vi "CD Init_Prepare Inline Data_Fill In BC part of Frame Descriptor.vi"(11 "message":T5 {"Timestamp Channel Data Reference" format="%.0x"; "Status Channel Data Refs" format="%.0x"; "Words Item Refs" format="%.0x"; "Words Block Data Refs"."Data Reference" format="%.0x"}) -> (3 "BC Frame Descriptor":T1 {"Status Channel Refs" format="%.0x"; "Words Block Data Refs"."Data Reference" format="%.0x"; "Timestamp Channel Data Reference" format="%.0x"})   [LabVIEW 2017, in "Ballard MIL-1553 Engine.lvlib"]
uses:
  Ballard MIL-1553 Engine.lvlib
  Shared/Controls and Global/RT Message.ctl
  Shared/Controls and Global/RT messageType.ctl
  Shared/Controls and Global/RT CWD1.ctl
  Shared/Controls and Global/RT CWD2.ctl
  <vilib>/NI Veristand/Custom Device API/Data Reference.ctl
  <vilib>/NI Veristand/Custom Device API/Custom Device Item Ref.ctl
  <vilib>/NI Veristand/Custom Device API/Block Data Reference.ctl
  Controls/RT Inline Frame Descriptor_BC.ctl
  <vilib>/NI VeriStand/Custom Device API/Custom Device API.lvlib
  Shared/Ballard 1553 Shared.lvlib
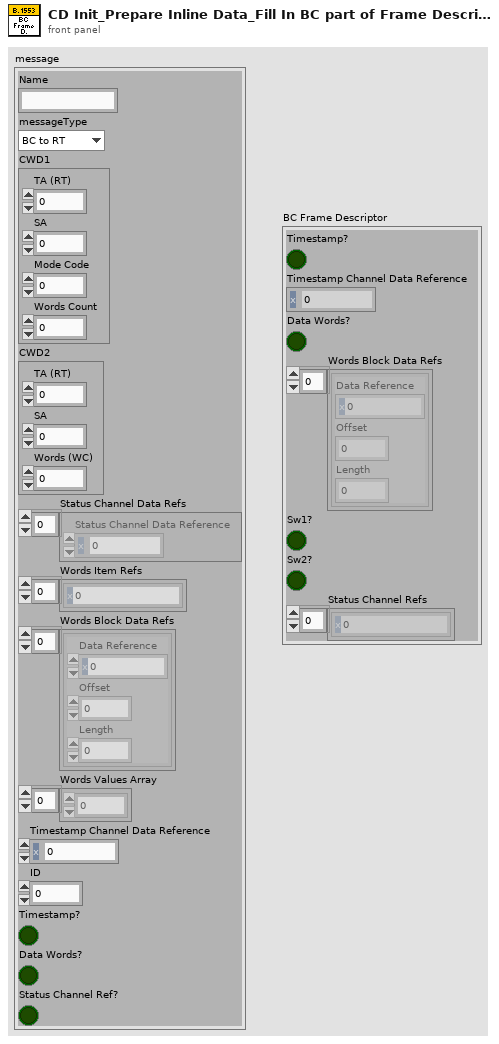
[diagram p1: front panel]
types:
  T1 = typedef "Ballard MIL-1553 Engine.lvlib/RT Inline Frame Descriptor_BC.ctl" = cluster{"Timestamp?":bool, "Timestamp Channel Data Reference":T2, "Data Words?":bool, "Words Block Data Refs":T3[], "Sw1?":bool, "Sw2?":bool, "Status Channel Refs":T4[]}
  T2 = typedef "Custom Device API.lvlib/Data Reference.ctl" = i32
  T3 = typedef "Custom Device API.lvlib/Block Data Reference.ctl" = cluster{"Data Reference":T2, "Offset":u64, "Length":u64}
  T4 = typedef "Custom Device API.lvlib/Custom Device Item Ref.ctl" = u64
  T5 = typedef "Ballard 1553 Shared.lvlib/RT Message.ctl" = cluster{"Name":string, "messageType":T6, "CWD1":T7, "CWD2":T8, "Status Channel Data Refs":T2[], "Words Item Refs":T4[], "Words Block Data Refs":T3[], "Words Values Array":u16[], "Timestamp Channel Data Reference":T2, "ID":i32, "Timestamp?":bool, "Data Words?":bool, "Status Channel Ref?":bool}
  T6 = typedef "Ballard 1553 Shared.lvlib/RT messageType.ctl" = enum16{"BC to RT", "RT to BC", "RT to RT", "MC (Rx)", "MC (Tx)"}
  T7 = typedef "Ballard 1553 Shared.lvlib/RT CWD1.ctl" = cluster{"TA (RT)":i8, "SA":i8, "Mode Code":i8, "Words Count":i8}
  T8 = typedef "Ballard 1553 Shared.lvlib/RT CWD2.ctl" = cluster{"TA (RT)":i8, "SA":i8, "Words (WC)":i8}
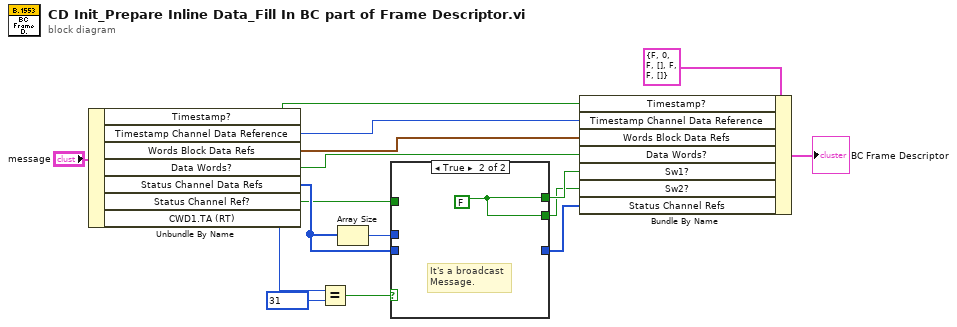
[diagram p0: block diagram]
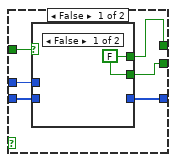
[diagram p2: hidden frame]
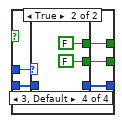
[diagram p3: hidden frame]
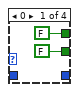
[diagram p4: hidden frame]
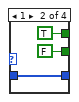
[diagram p5: hidden frame]
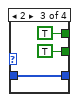
[diagram p6: hidden frame]
diagram:
  n1 = Unbundle By Name("message") -> ("Timestamp?"=w5:bool, "Timestamp Channel Data Reference"=w13:T2, "Words Block Data Refs"=w12:T3[], "Data Words?"=w3:bool, "Status Channel Data Refs"=w4:T2[], "Status Channel Ref?"=w1:bool, "CWD1.TA (RT)"=w2:i8)
  n2 = Equal?(x=w2, y=i8 31) -> (x = y?=w6:bool)
  n3 = Array Size(array=w4) -> (size(s)=w11:i32)
  n4 = case shown="True" w6 {
    tunnel: w11 -> [w22 _]
    tunnel: [w21 w39] -> w10
    tunnel: [w20 w39] -> w9
    tunnel: w4 -> [w19 _]
    tunnel: [w18 _] -> w8
    tunnel: w1 -> [w17 _]
    frame False {
      n5 = case shown="False" w17 {
        tunnel: w22 -> [_ w28]
        tunnel: [w23 w27] -> w21
        tunnel: [w23 w26] -> w20
        tunnel: w19 -> [_ w25]
        tunnel: [_ w24] -> w18
        frame False {
          w23 = FALSE
        }
        frame True {
          n6 = case shown="3, Default" w28 {
            tunnel: [FALSE TRUE TRUE FALSE] -> w27
            tunnel: [FALSE FALSE TRUE FALSE] -> w26
            tunnel: w25 -> [_ w31 w34 _]
            tunnel: [_ w31 w34 _] -> w24
            frame 0 {
            }
            frame 1 {
            }
            frame 2 {
            }
            frame 3, Default {
            }
          }
        }
      }
    }
    frame True {
      w39 = FALSE
      # "It's a broadcast\nMessage."
    }
  }
  n7 = Bundle By Name(cluster=T1 {"Timestamp?"=FALSE, "Timestamp Channel Data Reference"=0, "Data Words?"=FALSE, "Words Block Data Refs"=[], "Sw1?"=FALSE, "Sw2?"=FALSE, "Status Channel Refs"=[]} ("BC"), "Timestamp?"=w5, "Timestamp Channel Data Reference"=w13, "Words Block Data Refs"=w12, "Data Words?"=w3, "Sw1?"=w10, "Sw2?"=w9, "Status Channel Refs"=w8) -> (→"BC Frame Descriptor":T1)
